vi "Publish Discovered Nodes.vi"(8 "error in":errorcluster, 11 "Interactor in":refnum<class "Interactor.lvclass">) -> (0 "error out":errorcluster, 3 "Interactor out":refnum<class "Interactor.lvclass">)   [LabVIEW 2024, in "Interactor.lvlib" / "Interactor.lvclass"]
uses:
  Interactor.lvclass
  Interactor.lvclass/Interactor.ctl
  CANopen 2/Node States.ctl
  Example/Home Messages/Populate Nodes List Msg/Populate Nodes List Msg.lvclass/Populate Nodes List Msg.ctl
  <vilib>/ActorFramework/Message Enqueuer/Message Enqueuer.lvclass/Message Enqueuer.ctl
  <vilib>/ActorFramework/Message Enqueuer/Enqueue.vi
  Example/Home Messages/Populate Nodes List Msg/Populate Nodes List Msg.lvclass
  C:/Program Files/National Instruments/LabVIEW 2024/vi.lib/ActorFramework/Message/Message.lvclass
  <vilib>/Utility/LVClass/Get LV Class Name.vi
  <resource>/AFDebug/Generate Trace for Message.vi
  <vilib>/ActorFramework/Message Priority Queue/Priority Enqueue.vi
  CANopen Master/CANopen Master.lvclass
  CANopen Master.lvlib
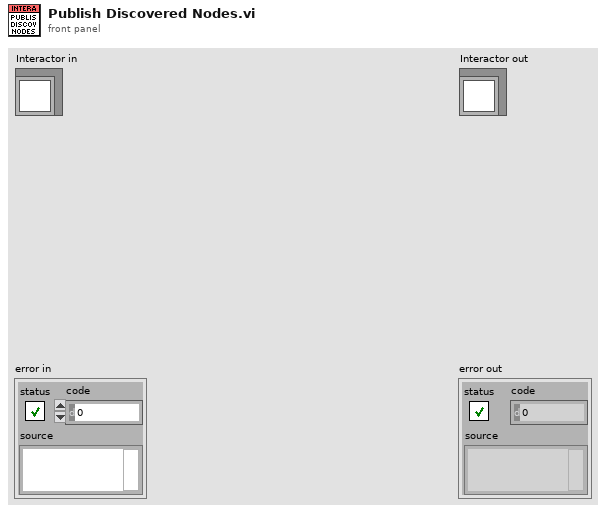
[diagram p1: front panel]
types:
  T1 = typedef "CANopen Master.lvlib/Node States.ctl" = map{u8, string}
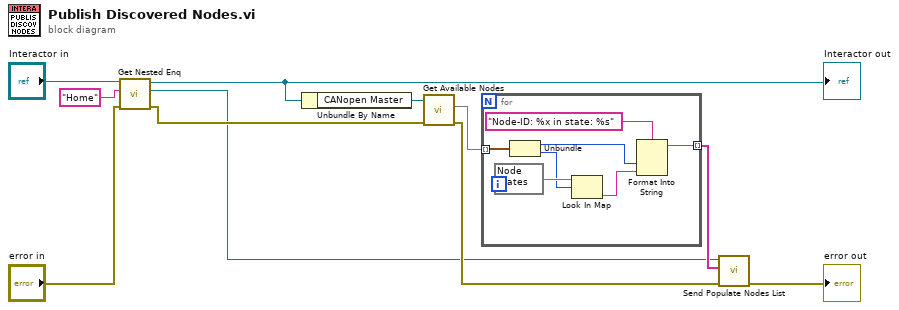
[diagram p0: block diagram]
diagram:
  n1 = call "Get Nested Enq.vi"("error in"="error in", "Ident"="Home", "Interactor in"="Interactor in") -> ("error out"=w2:errorcluster, "Enq"=w1:refnum<class "Message Enqueuer.lvclass">, "Interactor out"=w8:refnum<class "Interactor.lvclass">)  [unwired: 6 in]
  "Interactor out" <- w8
  n2 = Unbundle By Name(w8) -> ("CANopen Master"=w7:refnum<class "CANopen Master.lvclass">)
  n3 = call "Get Available Nodes.vi"("error in"=w2, "CANopen Master in"=w7) -> ("error out"=w5:errorcluster, "Nodes"=w6:map{u8, u8})  [unwired: 7 in, 1 out]
  n4 = for {
    tunnel: w6 -> [w18] mode=indexing
    tunnel: [w15] -> w4 mode=indexing
    n5 = Unbundle(w18) -> ("Node-ID"=w16:u8, "State"=w13:u8)
    n6 = Look In Map(map=T1 {0="Boot-up", 4="Stopped", 5="Operational", 127="Pre-operational"} ("Node States"), key=w13) -> (value=w12:string)  [unwired: 1 in, 1 out]
    n7 = Format Into String(format string="Node-ID: %x in state: %s", w16, w12) -> (resulting string=w15:string)  [unwired: 2 in, 1 out]
  }
  n8 = call "Send Populate Nodes List.vi"("error in (no error)"=w5, "Nodes"=w4, "Message Enqueuer"=w1) -> ("error out"=→"error out":errorcluster)  [unwired: 7 in, 1 out]
